vi "statusTank.vi"(1 "Value":dbl) -> (0 "vi reference":refnum<vi>)   [LabVIEW 2010]
panel:
  out "Tank":dbl(slide) min=0.0 max=100.0 step=1.0 scale=0.0..100.0
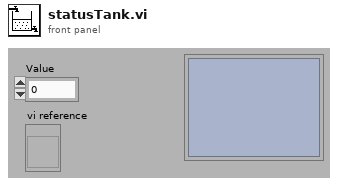
[diagram p1: front panel]
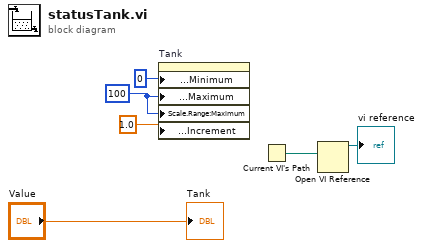
[diagram p0: block diagram]
diagram:
  w5 = 100
  n1 = property on="Tank" class="Slide (strict)"("Data Entry Limits:Minimum"=0, "Data Entry Limits:Maximum"=w5, "Scale.Range:Maximum"=w5, "Data Entry Limits:Increment"=1.0 ("Data Range:Increment")) -> ()  [unwired: 2 in, 2 out]
  n2 = Current VI's Path() -> (path=w2:path)
  n3 = Open VI Reference(vi path=w2) -> (vi reference=→"vi reference":refnum<vi>)  [unwired: 5 in, 1 out]
  "Tank" <- "Value"
